vi "Read Serial Device.lvclass.vi"(8 "error in (no error)":errorcluster, 11 "UI ACTOR in":refnum<class "UI ACTOR.lvclass">) -> (0 "error out":errorcluster, 2 "Serial Device.lvclass":refnum<class "Serial Device.lvclass">, 3 "UI ACTOR out":refnum<class "UI ACTOR.lvclass">)   [LabVIEW 2020, in "UI ACTOR.lvlib" / "UI ACTOR.lvclass"]
uses:
  UI ACTOR.lvclass
  HAL/Proyecto-Final/Abstract/Serial Device/Serial Device.lvclass
  UI ACTOR.lvclass/UI ACTOR.ctl
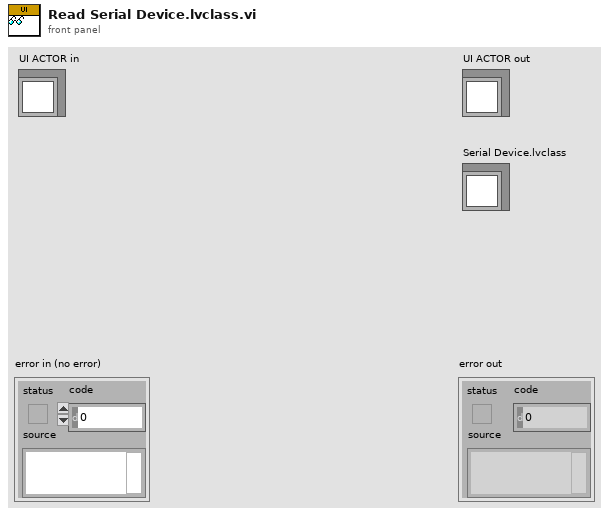
[diagram p1: front panel]
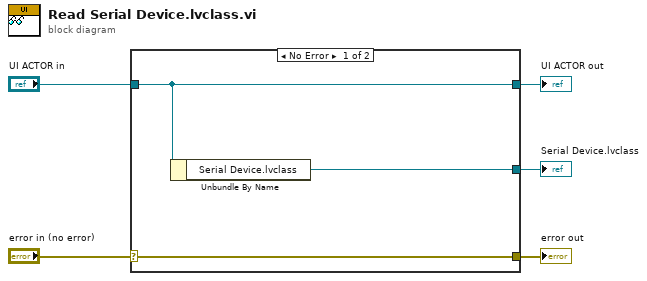
[diagram p0: block diagram]
diagram:
  n1 = case shown="No Error" "error in (no error)" {
    selector: "error in (no error)" -> [w8 w9]
    tunnel: [w8 w9] -> w4
    tunnel: [w7 w10] -> w2
    tunnel: "UI ACTOR in" -> [w7 w10]
    tunnel: [w6 _] -> w1
    frame No Error {
      n2 = Unbundle By Name(w7) -> ("Serial Device.lvclass"=w6:refnum<class "Serial Device.lvclass">)
    }
    frame Error {
    }
  }
  "error out" <- w4
  "UI ACTOR out" <- w2
  "Serial Device.lvclass" <- w1
